vi "Seq Dialog Vent AP test.vi"(8 "Segment Data":T1) -> (0 "Step Hisitory":string[](array[string]), 2 "Segment Data 2":T1)   [LabVIEW 2018]
uses:
  type defs/Sequence Info.ctl
  type defs/Vent AP Limts Seq.ctl
panel:
  in  "End Sample":dbl
  in  "Start Sample":dbl
  in  "Overall Max":dbl
  in  "Overall Min":dbl
  out "String 2":string="Pre Run Station - Glass - Vent Open"
  out "error out":errorcluster
  in  "Description":string
  in  "Save":bool
  in  "Cancel":bool
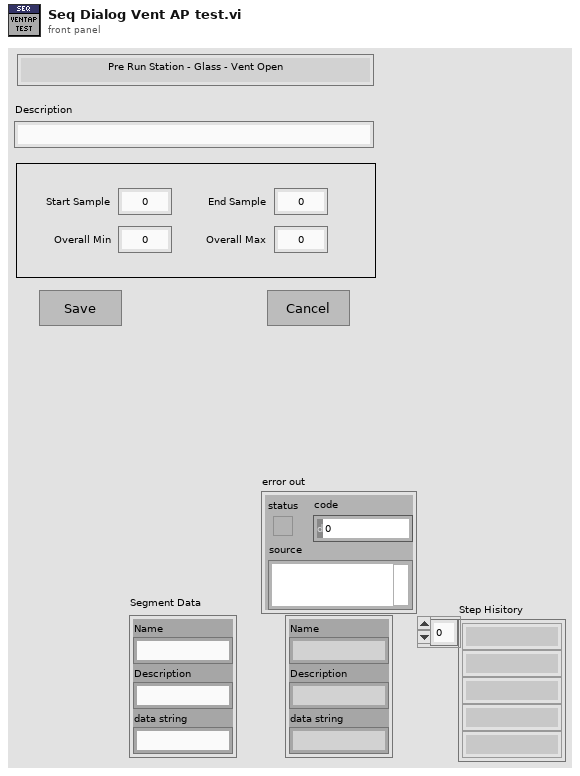
[diagram p1: front panel]
types:
  T1 = typedef "Sequence Info.ctl" = cluster{"Name":string, "Description":string, "data string":string}
  T2 = typedef "Vent AP Limts Seq.ctl" = cluster{"Overall Min":dbl, "Overall Max":dbl, "Truncation Start":dbl, "Truncation End":dbl}
  T3 = cluster{"Segment Data":T1, "Sun Shade Close Force":T2, "Old Data":string, "New Data":string}
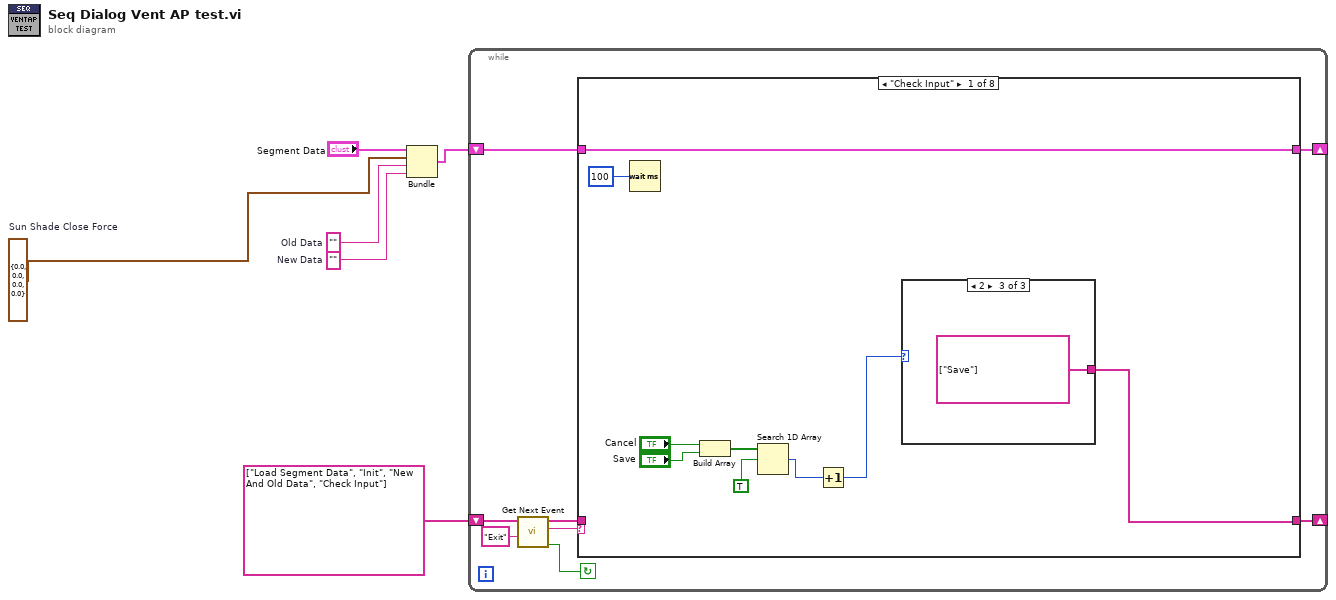
[diagram p0: block diagram]
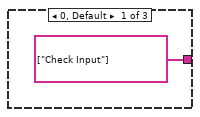
[diagram p2: hidden frame]
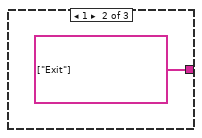
[diagram p3: hidden frame]
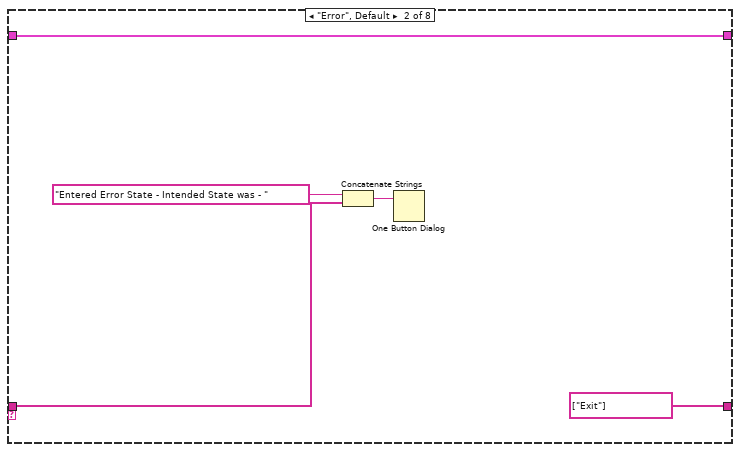
[diagram p4: hidden frame]
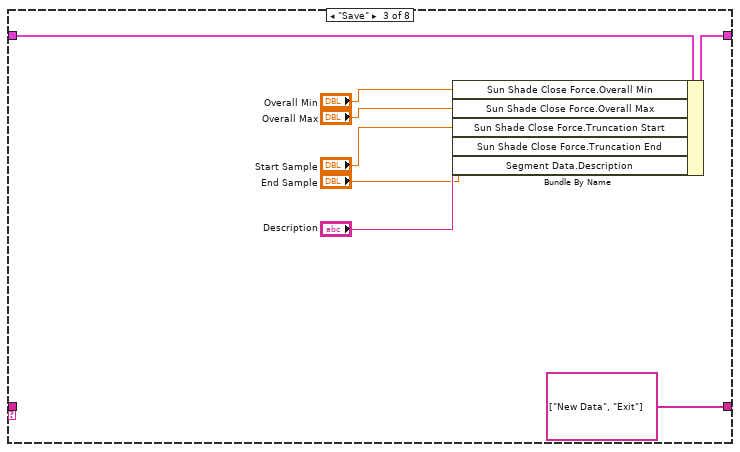
[diagram p5: hidden frame]
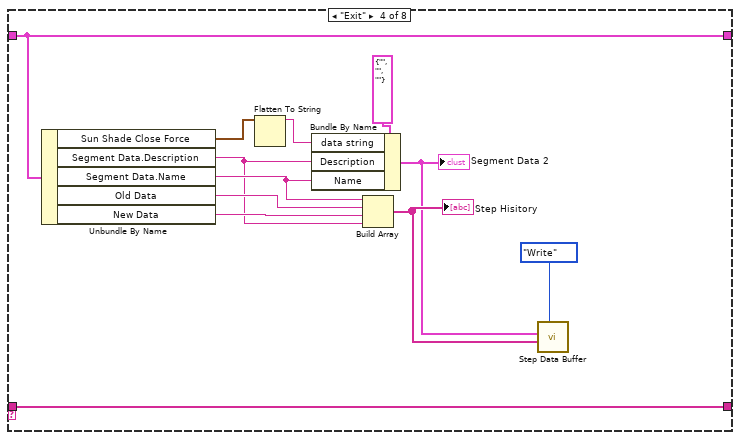
[diagram p6: hidden frame]
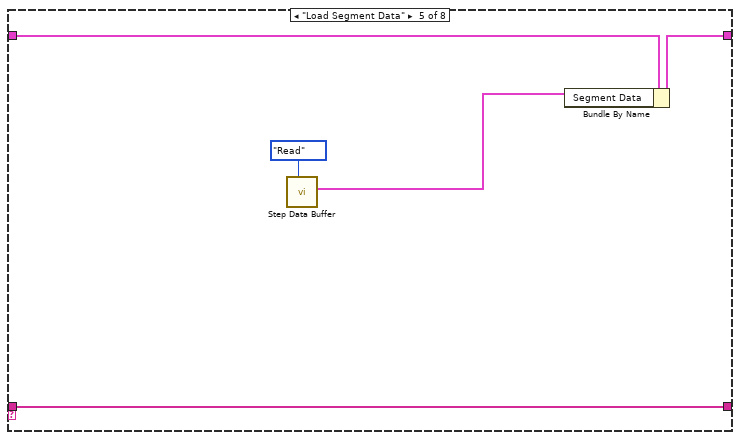
[diagram p7: hidden frame]
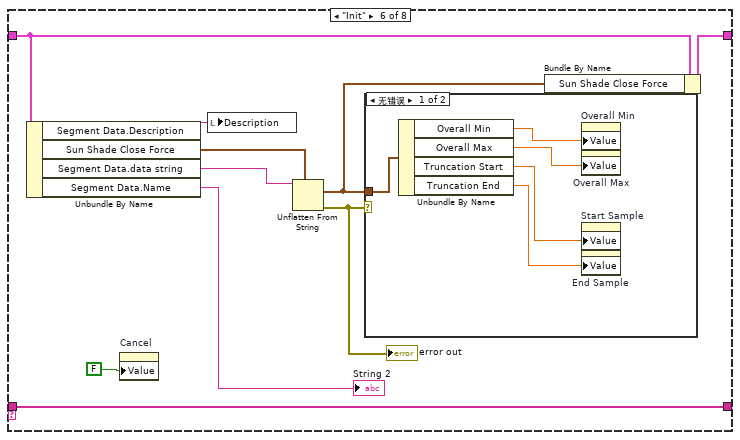
[diagram p8: hidden frame]
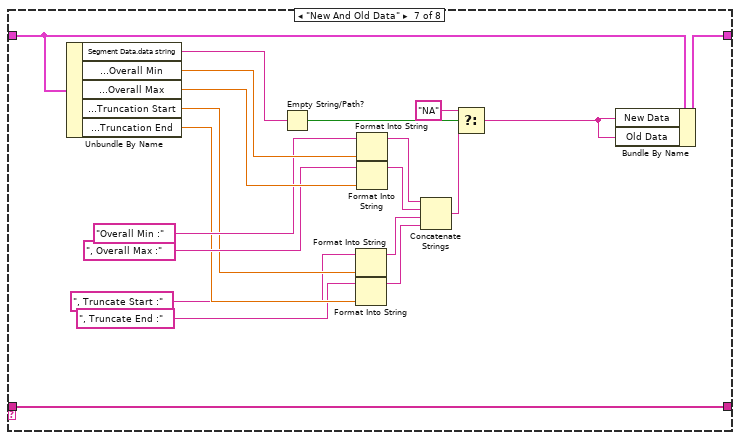
[diagram p10: hidden frame]
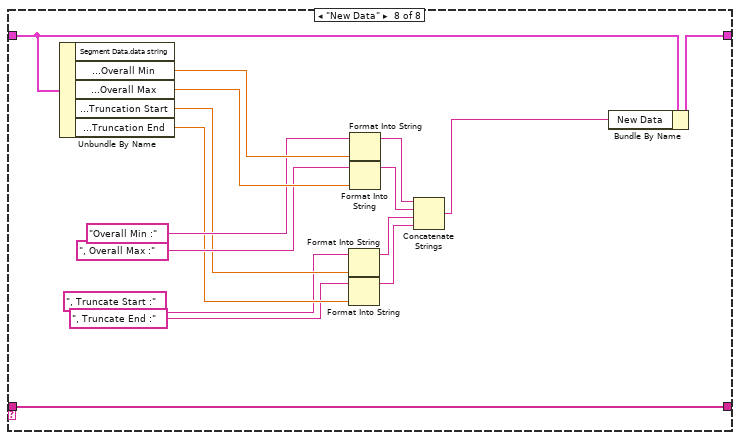
[diagram p11: hidden frame]
diagram:
  w1 = T2 {"Overall Min"=0.0, "Overall Max"=0.0, "Truncation Start"=0.0, "Truncation End"=0.0}  # Sun Shade Close Force
  w3 = ""  # New Data
  w4 = ""  # Old Data
  n1 = Bundle("Segment Data"="Segment Data", "Sun Shade Close Force"=w1, "Old Data"=w4, "New Data"=w3) -> (w5:T3)  [unwired: 1 in]
  n2 = while {
    shift-right: [w12] -> _
    shift-left: string[] ["Load Segment Data", "Init", "New And Old Data", "Check Input"] ("Event queue out") -> [w11]
    shift-right: [w7] -> _
    shift-left: w5 -> [w8]
    stop <- w10 continue-if-true
    n3 = call "Get Next Event.vi"("Exit Event"="Exit", "event queue in"=w11) -> ("Condition (Exit:F)"=w10:bool, "next event"=w14:string, "event queue out"=w13:string[])  [unwired: 3 in]
    n4 = case shown="\"Check Input\"" w14 {
      tunnel: w13 -> [_ w28 _ w51 w56 w66 w91 w95]
      tunnel: [w15 string[] ["Exit"] ("event queue out") string[] ["New Data", "Exit"] ("Event queue out") w51 w56 w66 w91 w95] -> w12
      tunnel: w8 -> [w18 w31 w38 w44 w53 w59 w79 w94]
      tunnel: [w18 w31 w37 w44 w52 w58 w78 w93] -> w7
      frame "Check Input" {
        n5 = Wait (ms)(milliseconds to wait=u32 100) -> ()  [unwired: 1 out]
        n6 = Build Array("Cancel", "Save") -> (w20:bool[])
        n7 = Search 1D Array(1D array=w20, element=TRUE) -> (index of element=w16:i32)  [unwired: 1 in]
        n8 = Increment(x=w16) -> (x+1=w17:i32)
        n9 = case shown="2" w17 {
          tunnel: [string[] ["Check Input"] ("Events to Insert") string[] ["Exit"] ("Events to Insert") string[] ["Save"] ("Events to Insert")] -> w15
          frame 0, Default {
          }
          frame 1 {
          }
          frame 2 {
          }
        }
      }
      frame "Error", Default {
        n10 = Concatenate Strings("Entered Error State - Intended State was - " ("string"), w28) -> (w29:string)
        n11 = One Button Dialog(message=w29) -> ()  [unwired: 1 in, 1 out]
      }
      frame "Save" {
        n12 = Bundle By Name(cluster=w38, "Sun Shade Close Force.Overall Min"="Overall Min", "Sun Shade Close Force.Overall Max"="Overall Max", "Sun Shade Close Force.Truncation Start"="Start Sample", "Sun Shade Close Force.Truncation End"="End Sample", "Segment Data.Description"="Description") -> (w37:T3)
      }
      frame "Exit" {
        n13 = Unbundle By Name(w44) -> ("Sun Shade Close Force"=w50:T2, "Segment Data.Description"=w40:string, "Segment Data.Name"=w45:string, "Old Data"=w47:string, "New Data"=w46:string)
        n14 = Flatten To String(anything=w50) -> (data string=w48:string)  [unwired: 3 in, 2 out]
        n15 = Bundle By Name(cluster=T1 {"Name"="", "Description"="", "data string"=""} ("Segment Data"), "data string"=w48, "Description"=w40, "Name"=w45) -> (w41:T1)
        "Segment Data 2" <- w41
        n16 = Build Array(w45, w47, w46, w40) -> (w42:string[])
        "Step Hisitory" <- w42
        n17 = call "Step Data Buffer.vi"("Mode"=enum16{"Init", "Read", "Write"}."Write", "Step Hisitory In"=w42, "Segment Data In"=w41) -> ()  [unwired: 4 in, 5 out]
      }
      frame "Load Segment Data" {
        n18 = call "Step Data Buffer.vi"("Mode"=enum16{"Init", "Read", "Write"}."Read") -> ("Segment Data Out"=w54:T1)  [unwired: 6 in, 4 out]
        n19 = Bundle By Name(cluster=w53, "Segment Data"=w54) -> (w52:T3)
      }
      frame "Init" {
        n20 = Unbundle By Name(w59) -> ("Segment Data.Description"=w61:string, "Sun Shade Close Force"=w64:T2, "Segment Data.data string"=w65:string, "Segment Data.Name"=→"String 2":string)
        n21 = property on="Cancel" class="Bool (严格)"("Value"=FALSE ("Cancel")) -> ()  [unwired: 2 in, 2 out]
        n22 = local write "Description"(w61) -> ()
        n23 = Unflatten From String(type=w64, binary string=w65) -> (value=w60:T2, error out=w63:errorcluster)  [unwired: 3 in, 1 out]
        "error out" <- w63
        n24 = case shown="无错误" w63 {
          tunnel: w60 -> [w71 _]
          frame No Error {
            n25 = Unbundle By Name(w71) -> ("Overall Min"=w70:dbl, "Overall Max"=w69:dbl, "Truncation Start"=w68:dbl, "Truncation End"=w67:dbl)
            n26 = property on="Overall Min" class="DigNum (严格)"("Value"=w70) -> ()  [unwired: 2 in, 2 out]
            n27 = property on="Overall Max" class="DigNum (严格)"("Value"=w69) -> ()  [unwired: 2 in, 2 out]
            n28 = property on="Start Sample" class="DigNum (严格)"("Value"=w68) -> ()  [unwired: 2 in, 2 out]
            n29 = property on="End Sample" class="DigNum (严格)"("Value"=w67) -> ()  [unwired: 2 in, 2 out]
          }
          frame Error {
          }
        }
        n30 = Bundle By Name(cluster=w59, "Sun Shade Close Force"=w60) -> (w58:T3)
      }
      frame "New And Old Data" {
        n31 = Unbundle By Name(w79) -> ("Segment Data.data string"=w90:string, "Sun Shade Close Force.Overall Min"=w85:dbl, "Sun Shade Close Force.Overall Max"=w83:dbl, "Sun Shade Close Force.Truncation Start"=w77:dbl, "Sun Shade Close Force.Truncation End"=w76:dbl)
        n32 = Empty String/Path?(string/path=w90) -> (empty?=w89:bool)
        n33 = Format Into String(initial string=", Truncate Start :" ("string"), w77) -> (resulting string=w75:string)  [unwired: 2 in, 1 out]
        n34 = Format Into String(initial string=", Truncate End :" ("string"), w76) -> (resulting string=w74:string)  [unwired: 2 in, 1 out]
        n35 = Format Into String(initial string="Overall Min :" ("string"), w85) -> (resulting string=w84:string)  [unwired: 2 in, 1 out]
        n36 = Format Into String(initial string=", Overall Max :" ("string"), w83) -> (resulting string=w82:string)  [unwired: 2 in, 1 out]
        n37 = Concatenate Strings(w84, w82, w75, w74) -> (w86:string)
        n38 = Select(t="NA", s=w89, f=w86) -> (s? t:f=w87:string)
        n39 = Bundle By Name(cluster=w79, "New Data"=w87, "Old Data"=w87) -> (w78:T3)
      }
      frame "New Data" {
        n40 = Unbundle By Name(w94) -> ("Sun Shade Close Force.Overall Min"=w107:dbl, "Sun Shade Close Force.Overall Max"=w105:dbl, "Sun Shade Close Force.Truncation Start"=w101:dbl, "Sun Shade Close Force.Truncation End"=w100:dbl)  [unwired: 1 out]
        n41 = Format Into String(initial string=", Truncate Start :" ("string"), w101) -> (resulting string=w99:string)  [unwired: 2 in, 1 out]
        n42 = Format Into String(initial string=", Truncate End :" ("string"), w100) -> (resulting string=w98:string)  [unwired: 2 in, 1 out]
        n43 = Format Into String(initial string="Overall Min :" ("string"), w107) -> (resulting string=w106:string)  [unwired: 2 in, 1 out]
        n44 = Format Into String(initial string=", Overall Max :" ("string"), w105) -> (resulting string=w104:string)  [unwired: 2 in, 1 out]
        n45 = Concatenate Strings(w106, w104, w99, w98) -> (w92:string)
        n46 = Bundle By Name(cluster=w94, "New Data"=w92) -> (w93:T3)
      }
    }
  }
